vi "Get_ODE_coefficients.vi"(11 "ODE Data in":T1={"Fluid Properties"={"Fluid"=enum."Air", "Temperature (K)"=0.0, "Pressure (Pa)"=0.0}, "SJ Geometry"={"Do (mm)"=0.0, "Ho (mm)"=0.0, "Dc (mm)"=0.0, "Hc (mm)"=0.0}, "Solution Controls"={"Simulation"=enum."Asymmetric", "Fixed Parameter"=enum."Pressure", "Model"=enum."Tang", "# time steps"=0, "# periods"=0, "Domain"=enum."Time", "Tolerance"=0.0, "STFT periods"=0}, "Misc Data"={"Amplitude Array"=[], "Freq jet"=0.0, "Coefficients"=[], "Nat Frequ"=1.205}, "Thermo and Transport Properties"={"nu"=0.0, "c"=0.0, "Pr"=0.0, "Cp"=0.0, "Cv"=0.0, "gamma"=0.0, "mu"=0.0, "rho"=0.0}, "LEM Output Data"={"X"=[], "times"=[], "|X|"=0.0, "PA X"=0.0}}) -> (3 "ODE Data out":T1={"Fluid Properties"={"Fluid"=enum."Air", "Temperature (K)"=0.0, "Pressure (Pa)"=0.0}, "SJ Geometry"={"Do (mm)"=0.0, "Ho (mm)"=0.0, "Dc (mm)"=0.0, "Hc (mm)"=0.0}, "Solution Controls"={"Simulation"=enum."Asymmetric", "Fixed Parameter"=enum."Pressure", "Model"=enum."Tang", "# time steps"=0, "# periods"=0, "Domain"=enum."Time", "Tolerance"=0.0, "STFT periods"=0}, "Misc Data"={"Amplitude Array"=[], "Freq jet"=0.0, "Coefficients"=[], "Nat Frequ"=1.205}, "Thermo and Transport Properties"={"nu"=0.0, "c"=0.0, "Pr"=0.0, "Cp"=0.0, "Cv"=0.0, "gamma"=0.0, "mu"=0.0, "rho"=0.0}, "LEM Output Data"={"X"=[], "times"=[], "|X|"=0.0, "PA X"=0.0}})   [LabVIEW 2012]
uses:
  SJ_ODE_Data.ctl
  Utilities/fluid_properties/fluid_types.ctl
  Model.ctl
  Utilities/fluid_properties/fluid_properties.ctl
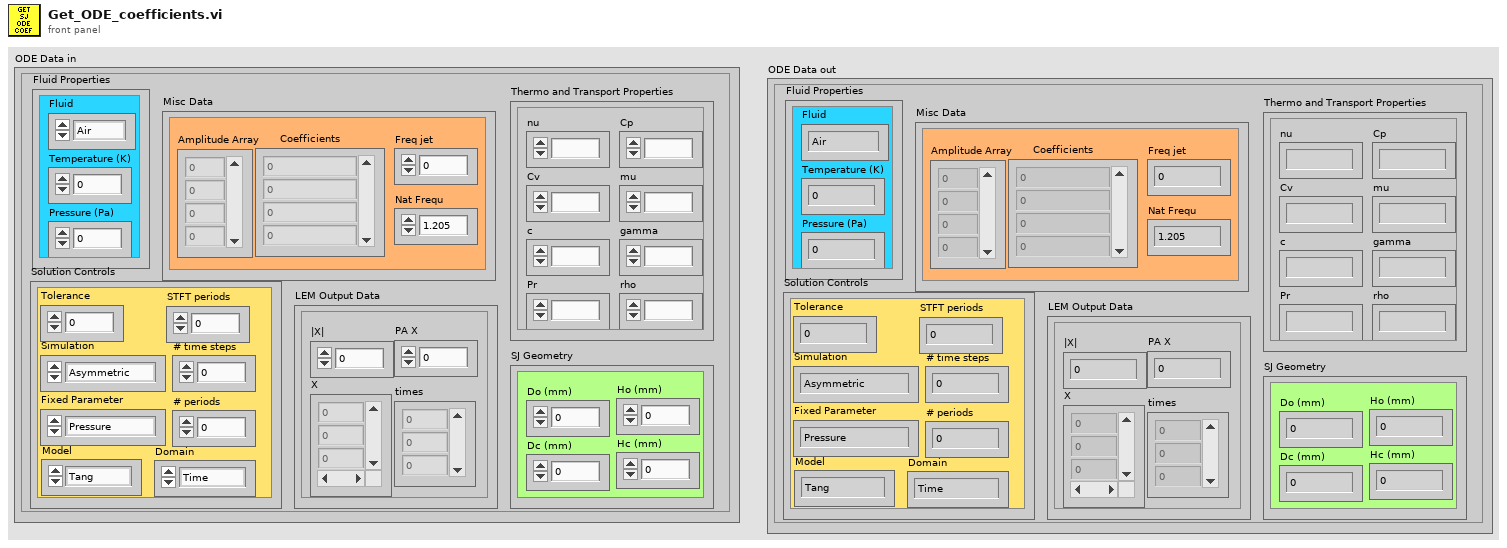
[diagram p1: front panel]
types:
  T1 = typedef "SJ_ODE_Data.ctl" = cluster{"Fluid Properties":cluster{"Fluid":T2, "Temperature (K)":dbl, "Pressure (Pa)":dbl}, "SJ Geometry":cluster{"Do (mm)":dbl, "Ho (mm)":dbl, "Dc (mm)":dbl, "Hc (mm)":dbl}, "Solution Controls":cluster{"Simulation":enum16{"Asymmetric", "Sinusoidal"}, "Fixed Parameter":enum16{"Pressure", "Displacement"}, "Model":T3, "# time steps":i32, "# periods":i32, "Domain":enum16{"Time", "Frequency"}, "Tolerance":dbl, "STFT periods":i32}, "Misc Data":cluster{"Amplitude Array":dbl[], "Freq jet":dbl, "Coefficients":dbl[], "Nat Frequ":dbl}, "Thermo and Transport Properties":T4, "LEM Output Data":cluster{"X":dbl[][], "times":dbl[], "|X|":dbl, "PA X":dbl}}
  T2 = typedef "fluid_types.ctl" = enum16{"Air", "Water"}
  T3 = typedef "Model.ctl" = enum16{"Tang", "Gallas", "Persoon"}
  T4 = typedef "fluid_properties.ctl" = cluster{"nu":dbl, "c":dbl, "Pr":dbl, "Cp":dbl, "Cv":dbl, "gamma":dbl, "mu":dbl, "rho":dbl}
  T5 = cluster{"Fluid":T2, "Temperature (K)":dbl, "Pressure (Pa)":dbl}
  T6 = cluster{"Do (mm)":dbl, "Ho (mm)":dbl, "Dc (mm)":dbl, "Hc (mm)":dbl}
  T7 = cluster{"Simulation":enum16{"Asymmetric", "Sinusoidal"}, "Fixed Parameter":enum16{"Pressure", "Displacement"}, "Model":T3, "# time steps":i32, "# periods":i32, "Domain":enum16{"Time", "Frequency"}, "Tolerance":dbl, "STFT periods":i32}
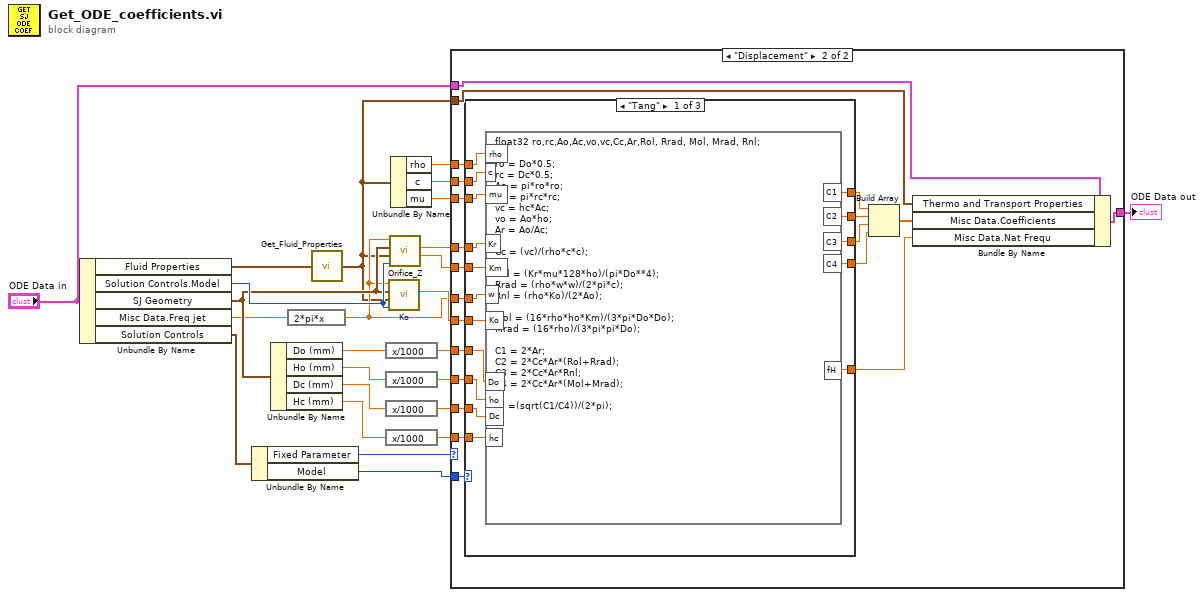
[diagram p0: block diagram]
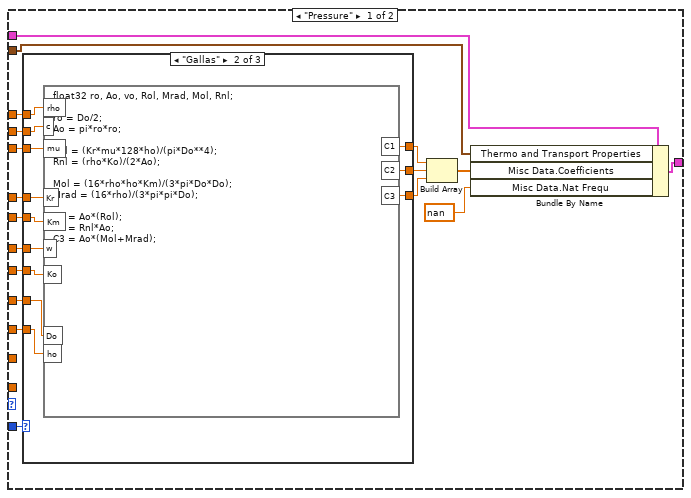
[diagram p2: hidden frame]
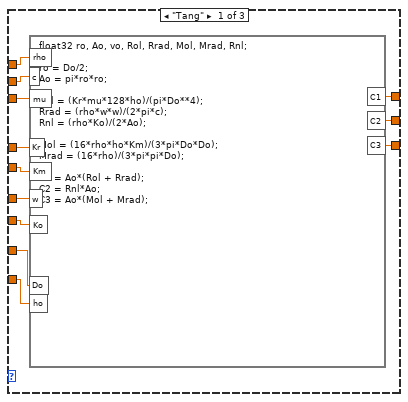
[diagram p3: hidden frame]
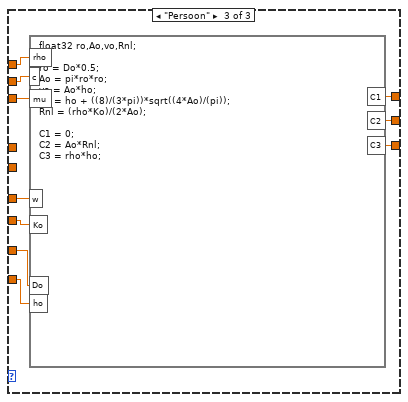
[diagram p4: hidden frame]
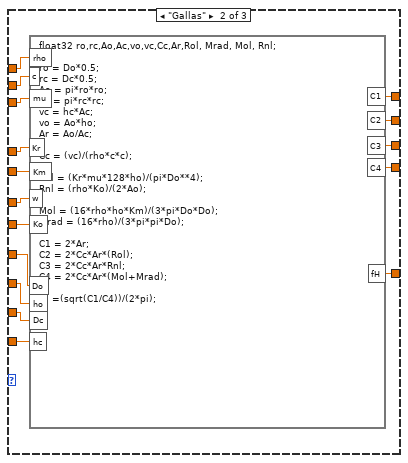
[diagram p5: hidden frame]
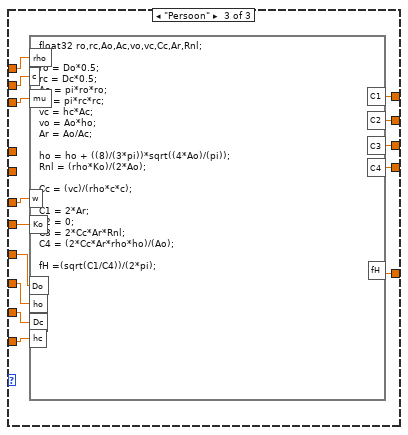
[diagram p6: hidden frame]
diagram:
  n1 = Unbundle By Name("ODE Data in") -> ("Fluid Properties"=w24:T5, "Solution Controls.Model"=w25:T3, "SJ Geometry"=w18:T6, "Misc Data.Freq jet"=w2:dbl, "Solution Controls"=w23:T7)
  n2 = Unbundle By Name(w23) -> ("Fixed Parameter"=w22:enum16{"Pressure", "Displacement"}, "Model"=w21:T3)
  n3 = Unbundle By Name(w18) -> ("Do (mm)"=w17:dbl, "Ho (mm)"=w15:dbl, "Dc (mm)"=w6:dbl, "Hc (mm)"=w5:dbl)
  n4 = expression code="2*pi*x"(w2) -> (w11:dbl)
  n5 = call "Get_Fluid_Properties.vi"("Fluid Properties"=w24) -> ("Thermo and Transport Properties"=w1:T4)  [unwired: 4 in]
  n6 = expression code="x/1000"(w17) -> (w8:dbl)
  n7 = expression code="x/1000"(w15) -> (w7:dbl)
  n8 = expression code="x/1000"(w6) -> (w4:dbl)
  n9 = expression code="x/1000"(w5) -> (w3:dbl)
  n10 = call "Ko.vi"("Model"=w25, "Thermo and Transport Properties"=w1, "SJ Geometry"=w18, "omega"=w11) -> ("Ko"=w16:dbl)  [unwired: 7 in]
  n11 = call "Orifice_Z.vi"("Model"=w25, "Thermo and Transport Properties"=w1, "SJ Geometry"=w18, "Omega"=w11) -> ("Km"=w9:dbl, "Kr"=w10:dbl)  [unwired: 5 in, 1 out]
  n12 = Unbundle By Name(w1) -> ("rho"=w14:dbl, "c"=w13:dbl, "mu"=w12:dbl)
  n13 = case shown="\"Displacement\"" w22 {
    tunnel: w21 -> [w43 w98]
    tunnel: "ODE Data in" -> [w42 w97]
    tunnel: [w41 w96] -> w19
    tunnel: w8 -> [w36 w91]
    tunnel: w16 -> [w35 w90]
    tunnel: w7 -> [w34 w89]
    tunnel: w14 -> [w33 w88]
    tunnel: w13 -> [w32 w87]
    tunnel: w12 -> [w31 w86]
    tunnel: w11 -> [w30 w85]
    tunnel: w10 -> [w29 w84]
    tunnel: w9 -> [w28 w83]
    tunnel: w4 -> [_ w82]
    tunnel: w3 -> [_ w81]
    tunnel: w1 -> [w27 w79]
    frame "Pressure" {
      n14 = case shown="\"Gallas\"" w43 {
        tunnel: [w55 w67 w77] -> w39
        tunnel: [w54 w66 w76] -> w38
        tunnel: [w53 w65 w75] -> w37
        tunnel: w36 -> [w52 w64 w74]
        tunnel: w35 -> [w51 w63 w73]
        tunnel: w34 -> [w50 w62 w72]
        tunnel: w33 -> [w49 w61 w71]
        tunnel: w32 -> [w48 w60 w70]
        tunnel: w31 -> [w47 w59 w69]
        tunnel: w30 -> [w46 w58 w68]
        tunnel: w29 -> [w45 w57 _]
        tunnel: w28 -> [w44 w56 _]
        frame "Tang" {
          n15 = formula code="float32 ro, Ao, vo, Rol, Rrad, Mol, Mrad, Rnl;\n\nro = Do/2;\nAo = pi*ro*ro;\n\nRol = (Kr*mu*128*ho)/(pi*Do**4);\nRrad = (rho*w*w)/(2*pi*c);\nRnl = (rho*Ko)/(2*Ao);\n\nMol = (16*rho*ho*Km)/(3*pi*Do*Do);\nMrad = (16*rho)/(3*pi*pi*Do);\n\nC1 = Ao*(Rol + Rrad);\nC2 = Rnl*Ao;\nC3 = Ao*(Mol + Mrad);"("Do"=w52, "Ko"=w51, "Kr"=w45, "ho"=w50, "rho"=w49, "c"=w48, "mu"=w47, "w"=w46, "Km"=w44) -> ("C1"=w55:dbl, "C2"=w54:dbl, "C3"=w53:dbl)
        }
        frame "Gallas" {
          n16 = formula code="float32 ro, Ao, vo, Rol, Mrad, Mol, Rnl;\n\nro = Do/2;\nAo = pi*ro*ro;\n\nRol = (Kr*mu*128*ho)/(pi*Do**4);\nRnl = (rho*Ko)/(2*Ao);\n\nMol = (16*rho*ho*Km)/(3*pi*Do*Do);\nMrad = (16*rho)/(3*pi*pi*Do);\n\nC1 = Ao*(Rol);\nC2 = Rnl*Ao;\nC3 = Ao*(Mol+Mrad);"("Do"=w64, "Ko"=w63, "Kr"=w57, "ho"=w62, "rho"=w61, "c"=w60, "mu"=w59, "w"=w58, "Km"=w56) -> ("C1"=w67:dbl, "C2"=w66:dbl, "C3"=w65:dbl)
        }
        frame "Persoon" {
          n17 = formula code="float32 ro,Ao,vo,Rnl;\n\nro = Do*0.5;\nAo = pi*ro*ro;\nvo = Ao*ho; \nho = ho + ((8)/(3*pi))*sqrt((4*Ao)/(pi));\nRnl = (rho*Ko)/(2*Ao);\n\nC1 = 0;\nC2 = Ao*Rnl;\nC3 = rho*ho;"("Do"=w74, "Ko"=w73, "ho"=w72, "rho"=w71, "c"=w70, "mu"=w69, "w"=w68) -> ("C1"=w77:dbl, "C2"=w76:dbl, "C3"=w75:dbl)
        }
      }
      n18 = Build Array(w39, w38, w37) -> (w40:dbl[])
      n19 = Bundle By Name(cluster=w42, "Thermo and Transport Properties"=w27, "Misc Data.Coefficients"=w40, "Misc Data.Nat Frequ"=nan) -> (w41:T1)
    }
    frame "Displacement" {
      n20 = case shown="\"Tang\"" w98 {
        tunnel: [w114 w130 w144] -> w94
        tunnel: [w113 w129 w143] -> w93
        tunnel: [w112 w128 w142] -> w92
        tunnel: w91 -> [w111 w127 w141]
        tunnel: w90 -> [w110 w126 w140]
        tunnel: w89 -> [w109 w125 w139]
        tunnel: w88 -> [w108 w124 w138]
        tunnel: w87 -> [w107 w123 w137]
        tunnel: w86 -> [w106 w122 w136]
        tunnel: w85 -> [w105 w121 w135]
        tunnel: w84 -> [w104 w120 _]
        tunnel: w83 -> [w103 w119 _]
        tunnel: w82 -> [w101 w117 w133]
        tunnel: w81 -> [w100 w116 w132]
        tunnel: [w102 w118 w134] -> w80
        tunnel: [w99 w115 w131] -> w78
        frame "Tang" {
          n21 = formula code="float32 ro,rc,Ao,Ac,vo,vc,Cc,Ar,Rol, Rrad, Mol, Mrad, Rnl;\n\nro = Do*0.5;\nrc = Dc*0.5;\nAo = pi*ro*ro;\nAc = pi*rc*rc;\nvc = hc*Ac;\nvo = Ao*ho; \nAr = Ao/Ac;\n\nCc = (vc)/(rho*c*c);\n\nRol = (Kr*mu*128*ho)/(pi*Do**4);\nRrad = (rho*w*w)/(2*pi*c);\nRnl = (rho*Ko)/(2*Ao);\n\nMol = (16*rho*ho*Km)/(3*pi*Do*Do);\nMrad = (16*rho)/(3*pi*pi*Do);\n\nC1 = 2*Ar;\nC2 = 2*Cc*Ar*(Rol+Rrad);\nC3 = 2*Cc*Ar*Rnl;\nC4 = 2*Cc*Ar*(Mol+Mrad);\n\nfH =(sqrt(C1/C4))/(2*pi);"("Do"=w111, "Ko"=w110, "Kr"=w104, "ho"=w109, "rho"=w108, "c"=w107, "mu"=w106, "w"=w105, "Km"=w103, "Dc"=w101, "hc"=w100) -> ("C1"=w114:dbl, "C2"=w113:dbl, "C3"=w112:dbl, "C4"=w102:dbl, "fH"=w99:dbl)
        }
        frame "Gallas" {
          n22 = formula code="float32 ro,rc,Ao,Ac,vo,vc,Cc,Ar,Rol, Mrad, Mol, Rnl;\n\nro = Do*0.5;\nrc = Dc*0.5;\nAo = pi*ro*ro;\nAc = pi*rc*rc;\nvc = hc*Ac;\nvo = Ao*ho; \nAr = Ao/Ac;\n\nCc = (vc)/(rho*c*c);\n\nRol = (Kr*mu*128*ho)/(pi*Do**4);\nRnl = (rho*Ko)/(2*Ao);\n\nMol = (16*rho*ho*Km)/(3*pi*Do*Do);\nMrad = (16*rho)/(3*pi*pi*Do);\n\nC1 = 2*Ar;\nC2 = 2*Cc*Ar*(Rol);\nC3 = 2*Cc*Ar*Rnl;\nC4 = 2*Cc*Ar*(Mol+Mrad);\n\nfH =(sqrt(C1/C4))/(2*pi);"("Do"=w127, "Ko"=w126, "Kr"=w120, "ho"=w125, "rho"=w124, "c"=w123, "mu"=w122, "w"=w121, "Km"=w119, "Dc"=w117, "hc"=w116) -> ("C1"=w130:dbl, "C2"=w129:dbl, "C3"=w128:dbl, "C4"=w118:dbl, "fH"=w115:dbl)
        }
        frame "Persoon" {
          n23 = formula code="float32 ro,rc,Ao,Ac,vo,vc,Cc,Ar,Rnl;\n\nro = Do*0.5;\nrc = Dc*0.5;\nAo = pi*ro*ro;\nAc = pi*rc*rc;\nvc = hc*Ac;\nvo = Ao*ho; \nAr = Ao/Ac;\n\nho = ho + ((8)/(3*pi))*sqrt((4*Ao)/(pi));\nRnl = (rho*Ko)/(2*Ao);\n\nCc = (vc)/(rho*c*c);\n\nC1 = 2*Ar;\nC2 = 0;\nC3 = 2*Cc*Ar*Rnl;\nC4 = (2*Cc*Ar*rho*ho)/(Ao);\n\nfH =(sqrt(C1/C4))/(2*pi);"("Do"=w141, "Ko"=w140, "ho"=w139, "rho"=w138, "c"=w137, "mu"=w136, "w"=w135, "Dc"=w133, "hc"=w132) -> ("C1"=w144:dbl, "C2"=w143:dbl, "C3"=w142:dbl, "C4"=w134:dbl, "fH"=w131:dbl)
        }
      }
      n24 = Build Array(w94, w93, w92, w80) -> (w95:dbl[])
      n25 = Bundle By Name(cluster=w97, "Thermo and Transport Properties"=w79, "Misc Data.Coefficients"=w95, "Misc Data.Nat Frequ"=w78) -> (w96:T1)
    }
  }
  "ODE Data out" <- w19
